vi "Verificarea defectiunilor.vi"() -> ()   [LabVIEW 2024]
panel:
  in  "Path":path
  in  "3D Picture 3":refnum<vi>(3d-picture)
  out "3D Picture 2":refnum<vi>(3d-picture)
  out "Piesa este defecta":bool
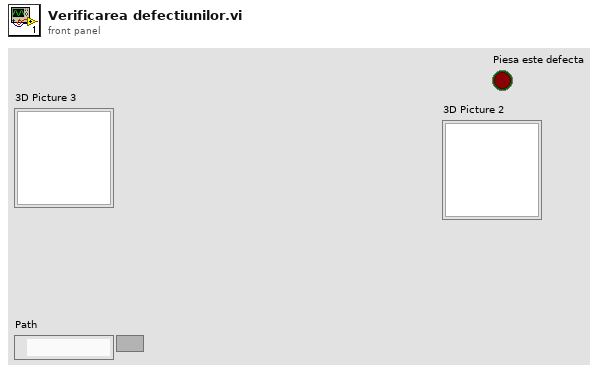
[diagram p1: front panel]
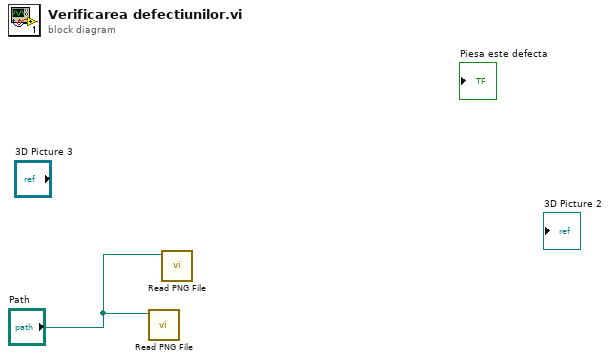
[diagram p0: block diagram]
diagram:
  n1 = call <vilib>:"Read PNG File.vi"("path to PNG file"="Path") -> ()  [unwired: 8 in, 3 out]
  n2 = call <vilib>:"Read PNG File.vi"("path to PNG file"="Path") -> ()  [unwired: 8 in, 3 out]
